vi "Schur Decomposition.vi"   [LabVIEW 2014, in "NI_AALPro.lvlib"]
doc: "Performs the Schur decomposition of a square matrix. Wire data to the <B>Input Matrix</B> input to determine the polymorphic instance to use or manually select the instance."
uses:
  NI_AALPro.lvlib
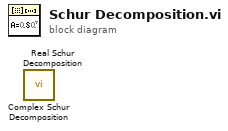
[diagram p0: block diagram]
diagram:
  n1 = call "Complex Schur Decomposition.vi"() -> ()  [unwired: 8 in, 4 out]
  n2 = call "Real Schur Decomposition.vi"() -> ()  [unwired: 8 in, 4 out]
